vi "System Actor Initialize.vi"(5 "Launching":bool=TRUE, 7 "Auto Dispose Ref":bool, 8 "error in (no error)":errorcluster, 10 "Root Actor Address":refnum<class "Mail Strategy.lvclass">, 11 "Device Connector in":refnum<class "Device Connector.lvclass">) -> (0 "error out":errorcluster, 2 "VI Refnum":refnum<vi>, 3 "Device Connector out":refnum<class "Device Connector.lvclass">)   [LabVIEW 2024, in "Device Connector.lvclass"]
uses:
  Device Connector.lvclass
  Ancestor Class/Messenger/Mail Strategy/Mail Strategy.lvclass
  Ancestor Class/Actor/System Actor/System Actor.lvclass
  Device Connector.lvclass/Device Connector.ctl
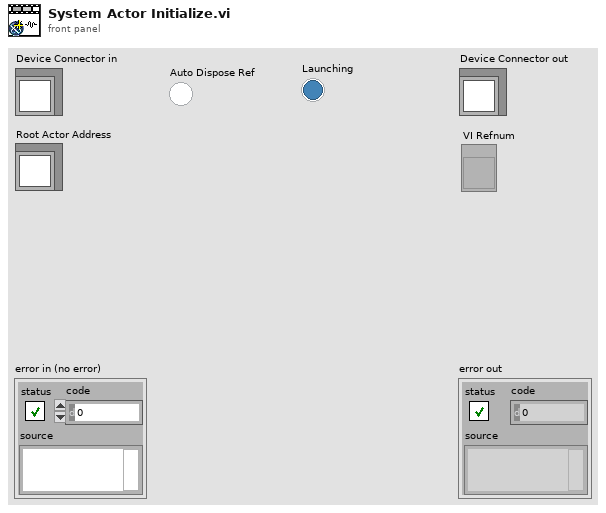
[diagram p1: front panel]
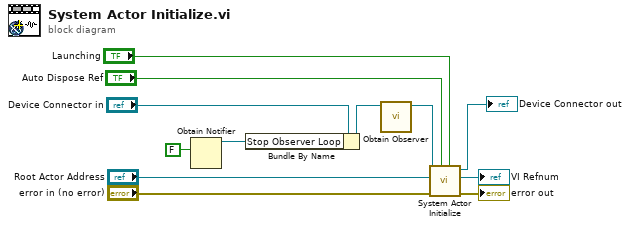
[diagram p0: block diagram]
diagram:
  n1 = Obtain Notifier(notification data type=FALSE) -> (notifier out=w6:refnum<notifier>)  [unwired: 3 in, 2 out]
  n2 = Bundle By Name(cluster="Device Connector in", "Stop Observer Loop"=w6) -> (w4:refnum<class "Device Connector.lvclass">)
  n3 = call-dynamic "Obtain Observer.vi"("Device Connector in"=w4) -> ("Device Connector out"=w3:refnum<class "Device Connector.lvclass">)  [unwired: 9 in, 1 out]
  n4 = call-parent "System Actor Initialize.vi"("Launching"="Launching", "Auto Dispose Ref"="Auto Dispose Ref", "error in (no error)"="error in (no error)", "Root Actor Address"="Root Actor Address", "System Actor in"=w3) -> ("error out"=→"error out":errorcluster, "VI Refnum"=→"VI Refnum":refnum<vi>, "System Actor out"=→"Device Connector out":refnum<class "Device Connector.lvclass">)  [unwired: 4 in]
